vi "Destroy Session.vi"(8 "error in (no error)":errorcluster, 11 "Session":T1) -> (0 "error out":errorcluster)   [LabVIEW 2023, in "LabVIEW Bodeplot Summit.lvlib"]
doc: "Destroy Measurement Link Session, Release hardware access"
uses:
  LabVIEW Bodeplot Summit.lvlib
  Session Info.ctl
  <vilib>/gRPC/LabVIEW gRPC Library/Shared/grpcId.ctl
  <vilib>/MeasurementLink/MeasurementLink Session Management Client/RPC Messages/ni_measurementlink_sessionmanagement_v1_ReserveSessionsResponse.ctl
  <vilib>/MeasurementLink/MeasurementLink Session Management Client/RPC Messages/ni_measurementlink_sessionmanagement_v1_SessionInformation.ctl
  <vilib>/MeasurementLink/MeasurementLink Session Management Client/RPC Messages/nidevice_grpc_Session.ctl
  <vilib>/MeasurementLink/MeasurementLink Session Management Client/RPC Messages/ni_measurementlink_sessionmanagement_v1_ChannelMapping.ctl
  <vilib>/MeasurementLink/MeasurementLink Discovery Client/MeasurementLink Discovery Client.lvlib
  <vilib>/MeasurementLink/MeasurementLink Session Management Client/MeasurementLink Session Management Client.lvlib
  <vilib>/gRPC/LabVIEW gRPC Library/grpc-lvsupport-release.lvlib
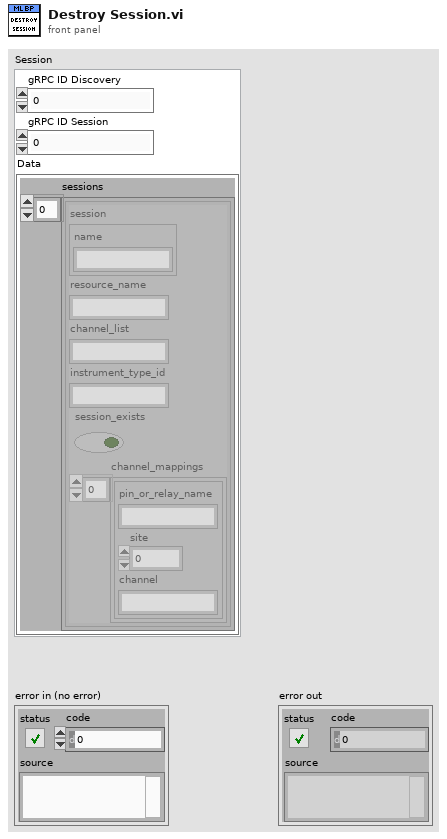
[diagram p1: front panel]
types:
  T1 = typedef "LabVIEW Bodeplot Summit.lvlib/Session Info.ctl" = cluster{"gRPC ID Discovery":T2, "gRPC ID Session":T2, "Data":T3}
  T2 = typedef "grpc-lvsupport-release.lvlib/grpcId.ctl" = u64
  T3 = typedef "MeasurementLink Session Management Client.lvlib/ni_measurementlink_sessionmanagement_v1_ReserveSessionsResponse.ctl" = cluster{"sessions":T4[]}
  T4 = typedef "MeasurementLink Session Management Client.lvlib/ni_measurementlink_sessionmanagement_v1_SessionInformation.ctl" = cluster{"session":T5, "resource_name":string, "channel_list":string, "instrument_type_id":string, "session_exists":bool, "channel_mappings":T6[]}
  T5 = typedef "MeasurementLink Session Management Client.lvlib/nidevice_grpc_Session.ctl" = cluster{"name":string}
  T6 = typedef "MeasurementLink Session Management Client.lvlib/ni_measurementlink_sessionmanagement_v1_ChannelMapping.ctl" = cluster{"pin_or_relay_name":string, "site":i32, "channel":string}
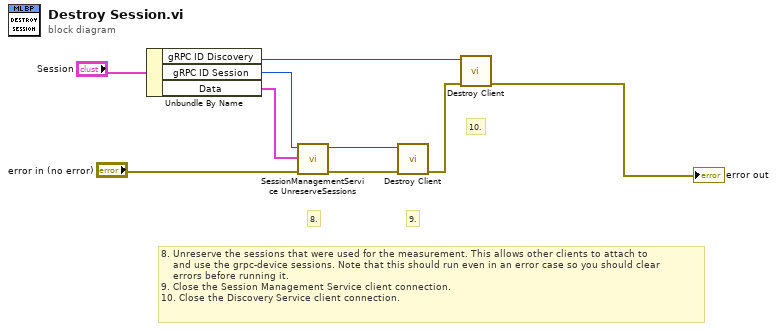
[diagram p0: block diagram]
diagram:
  # "8. Unreserve the sessions that were used for the measurement. This allows other clients to attach to\n    and use the grpc-device sessions. Note that this should run even in an error case so you should clear \n    errors before running it.\n9. Close the Session Management Service client connection.\n10. Close the Discovery Service client connection."
  # "10."
  # "9."
  # "8."
  n1 = Unbundle By Name("Session") -> ("gRPC ID Discovery"=w5:T2, "gRPC ID Session"=w4:T2, "Data"=w3:T3)
  n2 = call <vilib>:"SessionManagementService UnreserveSessions.vi"("error in"="error in (no error)", "Request Data"=w3, "gRPC ID"=w4) -> ("error out"=w7:errorcluster, "gRPC ID out"=w9:T2)  [unwired: 6 in, 1 out]
  n3 = call <vilib>:"Destroy Client.vi"("error in"=w7, "gRPC ID"=w9) -> ("error out"=w8:errorcluster)  [unwired: 9 in]
  n4 = call <vilib>:"Destroy Client.vi"("error in"=w8, "gRPC ID"=w5) -> ("error out"=→"error out":errorcluster)  [unwired: 9 in]
